vi "SetNumberArgument.vi"(2 "value":dbl, 3 "Argument":string, 4 "Argument List In":string[](array[string])) -> (0 "error out":errorcluster, 1 "Argument List Out":string[](array[string]))   [LabVIEW 2011]
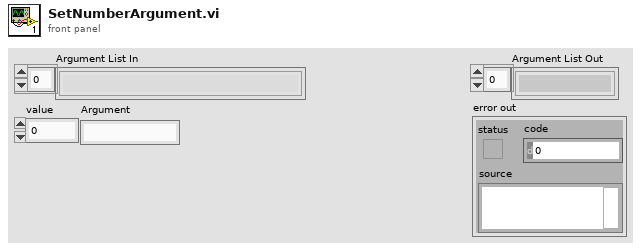
[diagram p1: front panel]
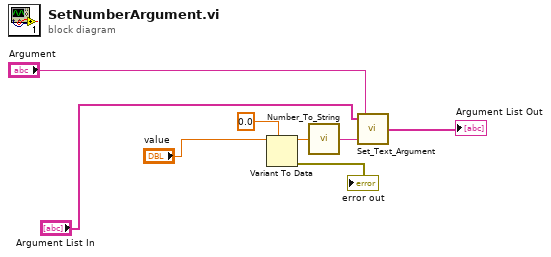
[diagram p0: block diagram]
diagram:
  n1 = Variant To Data(type=0.0, Variant="value") -> (data=w7:dbl, error out=→"error out":errorcluster)  [unwired: 1 in]
  n2 = call "Number_To_String.vi"("Number"=w7) -> ("String"=w6:string)
  n3 = call "Set_Text_Argument.vi"("Text"=w6, "Argument"="Argument", "Argument List In"="Argument List In") -> ("Argument List Out"=→"Argument List Out":string[])
